vi "GetMaxMin.vi"(8 "error in (no error)":errorcluster, 10 "Ignore Cal? (F)":bool, 11 "Strain in":refnum<class "Strain.lvclass">) -> (0 "error out":errorcluster, 1 "Min":cluster{"Value":dbl, "Text":string}, 2 "Max":cluster{"Value":dbl, "Text":string}, 3 "Strain out":refnum<class "Strain.lvclass">)   [LabVIEW 2012, in "Measurement Channels.lvlib" / "Strain.lvclass"]
uses:
  Strain.lvclass
  Strain.lvclass/Strain.ctl
  Class Channel/Read Device.vi
  <vilib>/Utility/TradDaqScaling.llb/Convert Strain Gauge Reading (scaler).vi
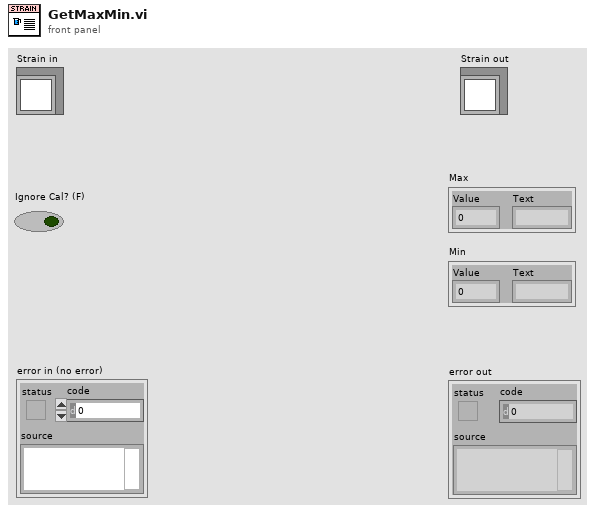
[diagram p1: front panel]
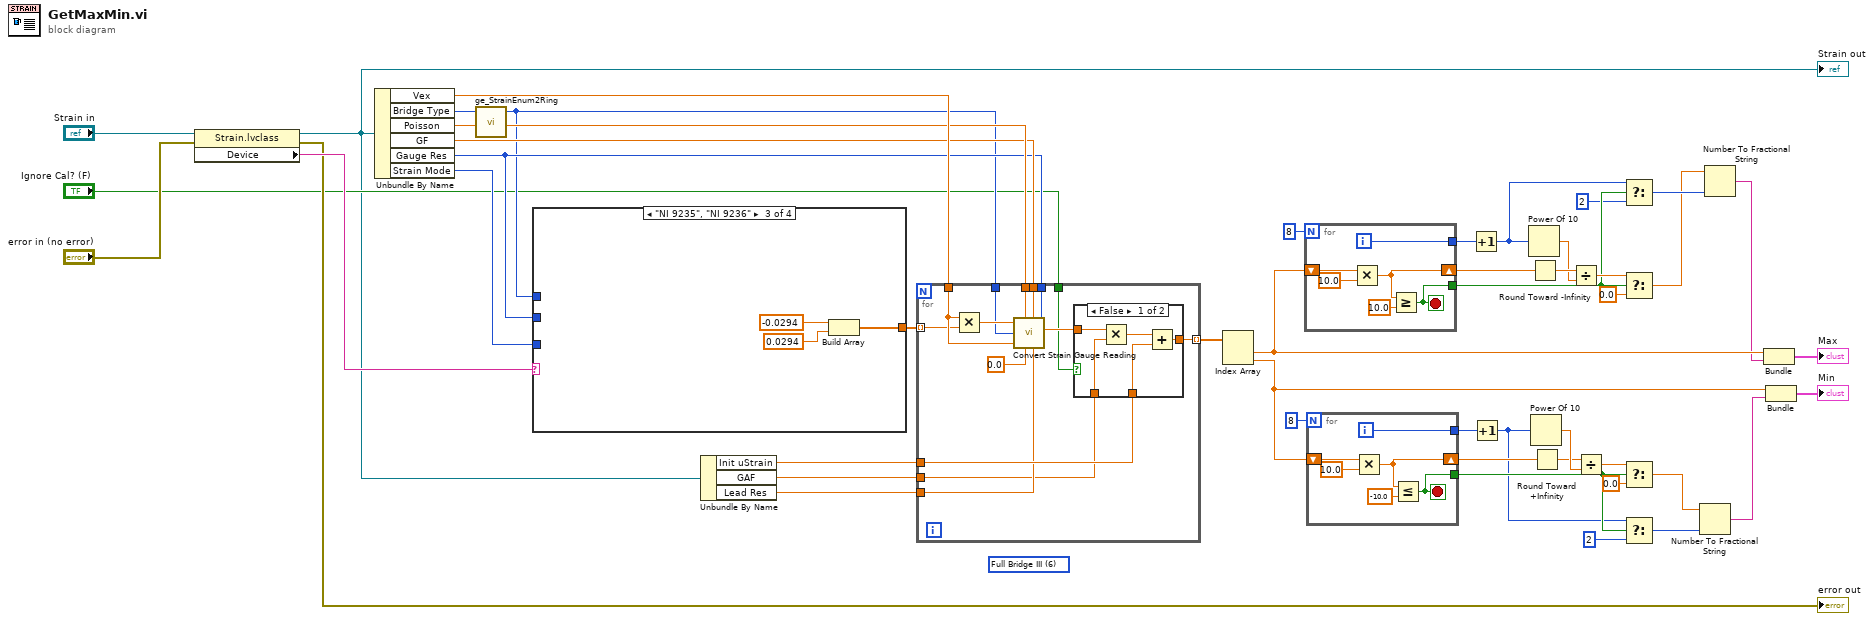
[diagram p0: block diagram]
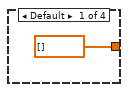
[diagram p3: hidden frame]
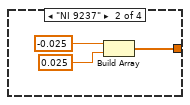
[diagram p4: hidden frame]
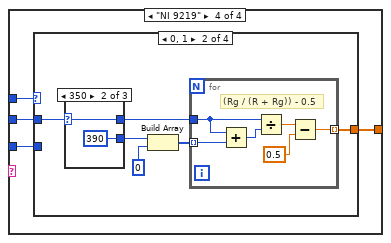
[diagram p5: hidden frame]
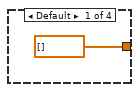
[diagram p6: hidden frame]
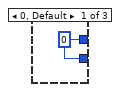
[diagram p7: hidden frame]
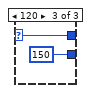
[diagram p8: hidden frame]
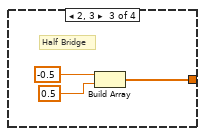
[diagram p9: hidden frame]
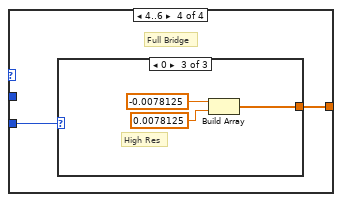
[diagram p10: hidden frame]
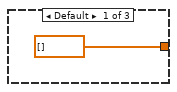
[diagram p11: hidden frame]
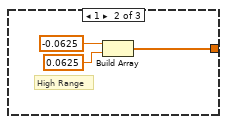
[diagram p12: hidden frame]
diagram:
  (unwired) u16 6 items=["Qtr Bridge I", "Qtr Bridge II", "Half Bridge I", "Half Bridge II", "Full Bridge I", "Full Bridge II", "Full Bridge III"] ("Bridge Configuration\n(3:Half Bridge II)")
  n1 = property class="Strain.lvclass"(reference="Strain in", error in="error in (no error)") -> (reference out=w1:refnum<class "Strain.lvclass">, error out=→"error out":errorcluster, "Device"=w16:string)
  "Strain out" <- w1
  n2 = Unbundle By Name(w1) -> ("Vex"=w48:dbl, "Bridge Type"=w47:u16, "Poisson"=w46:dbl, "GF"=w45:dbl, "Gauge Res"=w39:i32, "Strain Mode"=w40:u16)
  n3 = call "ge_StrainEnum2Ring.vi"("Bridge Type"=w47) -> ("Bridge Config Ring"=w28:u16)  [unwired: 4 in]
  n4 = case shown="\"NI 9235\", \"NI 9236\"" w16 {
    tunnel: [dbl[] [] w52 w55 w59] -> w44
    tunnel: w28 -> [_ _ _ w58]
    tunnel: w40 -> [_ _ _ w57]
    tunnel: w39 -> [_ _ _ w56]
    frame Default {
    }
    frame "NI 9237" {
      n5 = Build Array(-0.025, 0.025) -> (w52:dbl[])
    }
    frame "NI 9235", "NI 9236" {
      n6 = Build Array(-0.0294, 0.0294) -> (w55:dbl[])
    }
    frame "NI 9219" {
      n7 = case shown="0, 1" w58 {
        tunnel: [dbl[] [] w64 w80 w82] -> w59
        tunnel: w57 -> [_ _ _ w81]
        tunnel: w56 -> [_ w66 _ _]
        frame Default {
        }
        frame 0, 1 {
          n8 = case shown="350" w66 {
            selector: w66 -> [_ w75 w76]
            tunnel: [w73 390 ("y") 150 ("y")] -> w63
            tunnel: [w73 w75 w76] -> w61
            frame 0, Default {
              w73 = 0 ("Gauge Res")
            }
            frame 350 {
            }
            frame 120 {
            }
          }
          n9 = Build Array(w63, 0 ("Gauge Res")) -> (w65:i32[])
          n10 = for {
            tunnel: [w69] -> w64 mode=indexing
            tunnel: w61 -> [w68]
            tunnel: w65 -> [w67] mode=indexing
            # "(Rg / (R + Rg)) - 0.5"
            n11 = Add(x=w68, y=w67) -> (x+y=w70:i32)
            n12 = Divide(x=w68, y=w70) -> (x/y=w71:dbl)
            n13 = Subtract(x=w71, y=0.5) -> (x-y=w69:dbl)
          }
        }
        frame 2, 3 {
          # "Half Bridge"
          n14 = Build Array(-0.5, 0.5) -> (w80:dbl[])
        }
        frame 4..6 {
          # "Full Bridge"
          n15 = case shown="0" w81 {
            tunnel: [dbl[] [] w86 w89] -> w82
            frame Default {
            }
            frame 1 {
              # "High Range"
              n16 = Build Array(-0.0625, 0.0625) -> (w86:dbl[])
            }
            frame 0 {
              # "High Res"
              n17 = Build Array(-0.0078125, 0.0078125) -> (w89:dbl[])
            }
          }
        }
      }
    }
  }
  n18 = Unbundle By Name(w1) -> ("Init uStrain"=w17:dbl, "GAF"=w41:dbl, "Lead Res"=w42:dbl)
  n19 = for {
    tunnel: w48 -> [w97]
    tunnel: w46 -> [w102]
    tunnel: w45 -> [w101]
    tunnel: w39 -> [w100]
    tunnel: w17 -> [w99]
    tunnel: w28 -> [w91]
    tunnel: w44 -> [w96] mode=indexing
    tunnel: [w95] -> w43 mode=indexing
    tunnel: w42 -> [w94]
    tunnel: w41 -> [w92]
    tunnel: "Ignore Cal? (F)" -> [w90]
    n20 = Multiply(x=w97, y=w96) -> (x*y=w103:dbl)
    n21 = call-poly <vilib>:"Convert Strain Gauge Reading.vi"("Vsg (0.0)"=w103, "v (0.0)"=w102, "Bridge Configuration\n(3:Half Bridge II)"=w91, "Vex (3.33)"=w97, "Vinit (0.0)"=sgl 0.0, "GF (2.0)"=w101, "Rg (120)"=w100, "Rl (0.0)"=w94) -> ("Strain"=w93:sgl)  [unwired: 2 in]
    n22 = case shown="False" w90 {
      tunnel: w99 -> [w108 _]
      tunnel: [w107 w109] -> w95
      tunnel: w93 -> [w106 w109]
      tunnel: w92 -> [w105 _]
      frame False {
        n23 = Multiply(x=w106, y=w105) -> (x*y=w104:dbl)
        n24 = Add(x=w104, y=w108) -> (x+y=w107:dbl)
      }
      frame True {
      }
    }
  }
  n25 = Index Array(array=w43) -> (element #1=w10:dbl, element #2=w7:dbl)  [unwired: 2 in]
  n26 = for {
    N: 8 -> [_]
    tunnel: [w111] -> w29
    shift-right: [w112] -> w37
    shift-left: w10 -> [w115]
    tunnel: [w110] -> w25
    i -> [w111]
    stop <- w110 stop-if-true
    n27 = Multiply(x=w115, y=10.0) -> (x*y=w112:dbl)
    n28 = Greater Or Equal?(x=w112, y=10.0) -> (x >= y?=w110:bool)
  }
  n29 = for {
    N: 8 -> [_]
    tunnel: [w117] -> w30
    shift-right: [w118] -> w32
    shift-left: w7 -> [w121]
    tunnel: [w116] -> w20
    i -> [w117]
    stop <- w116 stop-if-true
    n30 = Multiply(x=w121, y=10.0) -> (x*y=w118:dbl)
    n31 = Less Or Equal?(x=w118, y=-10.0) -> (x <= y?=w116:bool)
  }
  n32 = Increment(x=w29) -> (x+1=w24:i32)
  n33 = Increment(x=w30) -> (x+1=w19:i32)
  n34 = Power Of 10(x=w24) -> (10^x=w35:dbl)
  n35 = Round Toward -Infinity(1:w37) -> (0:w36:dbl)
  n36 = Power Of 10(x=w19) -> (10^x=w34:dbl)
  n37 = Round Toward +Infinity(x=w32) -> (ceil(x): smallest int >= x=w33:dbl)
  n38 = Divide(x=w36, y=w35) -> (x/y=w27:dbl)
  n39 = Divide(x=w33, y=w34) -> (x/y=w21:dbl)
  n40 = Select(t=w24, s=w25, f=2) -> (s? t:f=w12:i32)
  n41 = Select(t=w27, s=w25, f=0.0) -> (s? t:f=w11:dbl)
  n42 = Select(t=w21, s=w20, f=0.0) -> (s? t:f=w5:dbl)
  n43 = Select(t=w19, s=w20, f=2) -> (s? t:f=w6:i32)
  n44 = Number To Fractional String(number=w5, precision (6)=w6) -> (F-format string=w4:string)  [unwired: 2 in]
  n45 = Number To Fractional String(number=w11, precision (6)=w12) -> (F-format string=w9:string)  [unwired: 2 in]
  n46 = Bundle("Strain"=w10, w9) -> (→"Max":cluster{"Strain":dbl, string})  [unwired: 1 in]
  n47 = Bundle("Strain"=w7, w4) -> (→"Min":cluster{"Strain":dbl, string})  [unwired: 1 in]
